vi "Split and merge.vi"(4 "DKE_Meaning":string="'A' leads letters; the Ancient Lord Leads and lords the entire world", 6 "Translation":string="'A' leads letters; the Ancient Lord Leads and lords the entire world", 7 "Index":string="அறத்துப்பால் - பாயிரம் - கடவுள் வாழ்த்து - ", 8 "DKT_Meaning":string="பகவன் முதற்றே உலகு.", 9 "Line 2":string="பகவன் முதற்றே உலகு.", 10 "Line1":string="அகர முதல எழுத்தெல்லாம் ஆதி", 11 "String In":string="\\par\r\n\r\n\\pard\\fi-2880\\li2880\\tx2880\\f2\\lang1097  \\f0  \\par\r\n\\u2990?\\u3009?\\u2965?\\u2984?\\u2965? \\u2984?\\u2975?\\u3021?\\u2986?\\u2980?\\u3009? \\u2984?\\u2975?\\u3021?\\u2986?\\u2985?\\u3021?\\u2993?\\u3009?\\par\r\n\\u2949?\\u2965?\\u2984?\\u2965? \\u2984?\\u2975?\\u3021?\\u2986?\\u2980?\\u3009?\\par\r\n\\b0\\f1\\fs36\\lang1033   \\par\r\nFriendship is not more smile on face\\par\r\nIt is the smiling heart's embrace\\par\r\n\\f2\\fs24\\lang1097   \\f0\\par\r\n\\u2986?\\u3006?\\u2994?\\u3021?- \\u2986?\\u3018?\\u2992?\\u3009?\\u2995?\\u3021?, \\u2951?\\u2991?\\u2994?\\u3021? - \\u2984?\\u2975?\\u3021?\\u2986?\\u3007?\\u2991?\\u2994?\\u3021?, \\u2949?\\u2980?\\u3007?\\u2965?\\u3006?\\u2992?\\u2990?\\u3021? - \\u2984?\\u2975?\\u3021?\\u2986?\\u3009? - ") -> (3 "String Output":string="\\par\r\n\\u2949?\\u2965?\\u2992? \\u2990?\\u3009?\\u2980?\\u2994? \\u2958?\\u2996?\\u3009?\\u2980?\\u3021?\\u2980?\\u3014?\\u2994?\\u3021?\\u2994?\\u3006?\\u2990?\\u3021? \\u2950?\\u2980?\\u3007?\\par\r\n\\u2986?\\u2965?\\u2997?\\u2985?\\u3021? \\u2990?\\u3009?\\u2980?\\u2993?\\u3021?\\u2993?\\u3015? \\u2953?\\u2994?\\u2965?\\u3009?.\\par\r\n\\u2949?\\u2965?\\u2984?\\u2965? \\u2984?\\u2975?\\u3021?\\u2986?\\u2980?\\u3009?\\par\r\n\\b0\\f1\\fs36\\lang1033   \\par\r\n'A' leads letters; the Ancient Lord \\par\r\nLeads and lords the entire world\\par\r\n\\f2\\fs24\\lang1097   \\f0\\par\r\n\\u2949?\\u2993?\\u2980?\\u3021?\\u2980?\\u3009?\\u2986?\\u3021?\\u2986?\\u3006?\\u2994?\\u3021? - \\u2986?\\u3006?\\u2991?\\u3007?\\u2992?\\u2990?\\u3021? - \\u2965?\\u2975?\\u2997?\\u3009?\\u2995?\\u3021? \\u2997?\\u3006?\\u2996?\\u3021?\\u2980?\\u3021?\\u2980?\\u3009? - ")   [LabVIEW 2019]
doc: "This VI is Developed by Anish Prabu T.\n\nCopyright © 2006, email:anishprabu243@yahoo.co.in.\nAll rights reserved."
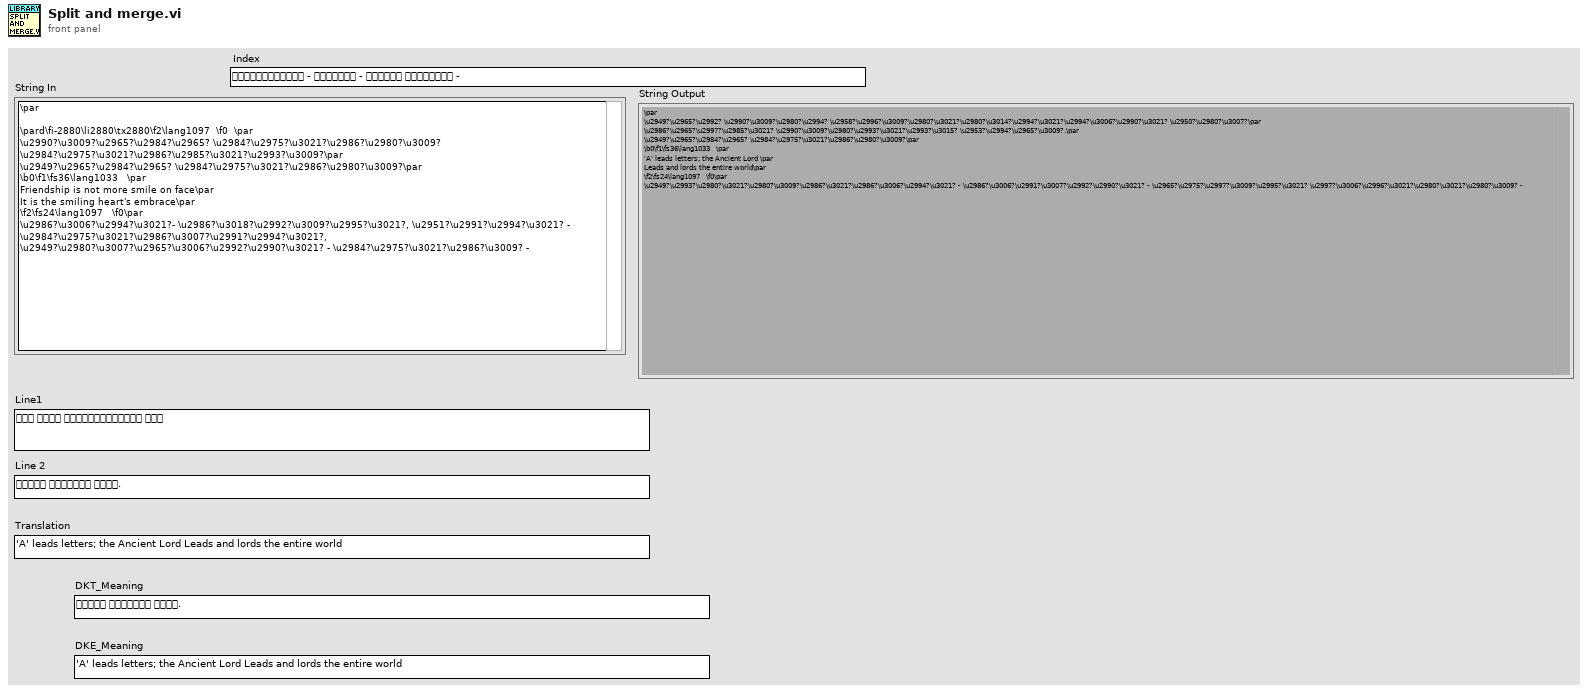
[diagram p1: front panel]
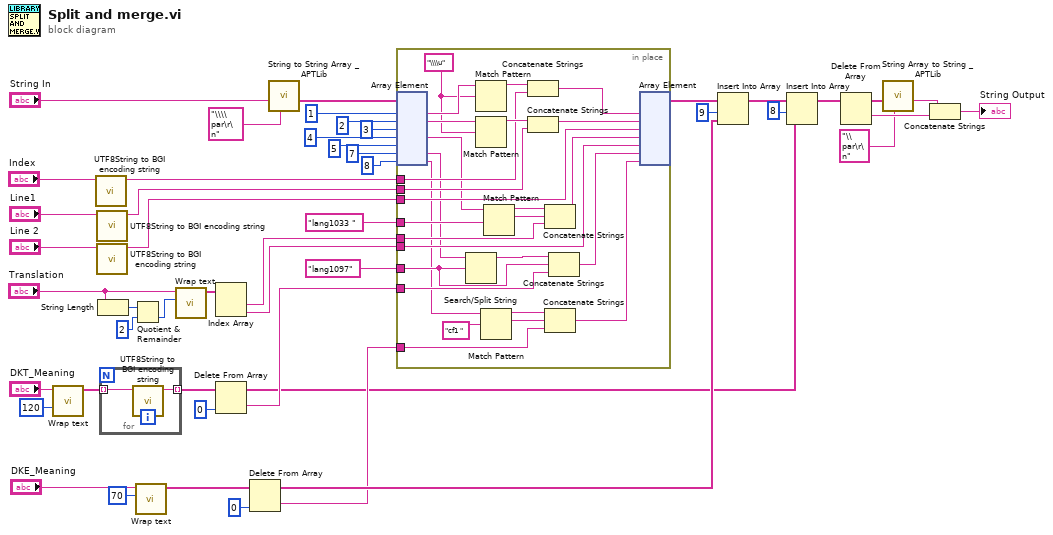
[diagram p0: block diagram]
diagram:
  n1 = call "Wrap text.vi"("Wrap Length"=120, "Text"="DKT_Meaning") -> ("Texts"=w25:string[])  [unwired: 9 in]
  n2 = call "UTF8String to BGI encoding string.vi"("Line1"="Index") -> ("String"=w37:string)  [unwired: 10 in]
  n3 = call "UTF8String to BGI encoding string.vi"("Line1"="Line1") -> ("String"=w35:string)  [unwired: 10 in]
  n4 = call "UTF8String to BGI encoding string.vi"("Line1"="Line 2") -> ("String"=w34:string)  [unwired: 10 in]
  n5 = String Length(string="Translation") -> (length=w12:i32)
  n6 = for {
    tunnel: w25 -> [w50] mode=indexing
    tunnel: [w49] -> w24 mode=indexing
    n7 = call "UTF8String to BGI encoding string.vi"("Line1"=w50) -> ("String"=w49:string)  [unwired: 10 in]
  }
  n8 = Quotient & Remainder(x=w12, y=2) -> (floor(x/y)=w10:i32)  [unwired: 1 out]
  n9 = call "Wrap text.vi"("Wrap Length"=70, "Text"="DKE_Meaning") -> ("Texts"=w14:string[])  [unwired: 9 in]
  n10 = call "Wrap text.vi"("Wrap Length"=w10, "Text"="Translation") -> ("Texts"=w9:string[])  [unwired: 9 in]
  n11 = Index Array(array=w9) -> (element #1=w8:string, element #2=w7:string)  [unwired: 2 in]
  n12 = Delete From Array(array=w24, index=0) -> (deleted portion=w6:string, array with subset deleted=w1:string[])  [unwired: 1 in]
  n13 = Delete From Array(array=w14, index=0) -> (deleted portion=w5:string, array with subset deleted=w18:string[])  [unwired: 1 in]
  n14 = call <userlib>:"String to String Array _APTLib.vi"("Seperator"="\\\\par\r\n", "String Input"="String In") -> ("String Array"=w32:string[])  [unwired: 8 in, 1 out]
  n15 = in-place {
    in-place-border: w37 -> [w69]
    in-place-border: w35 -> [w73]
    in-place-border: w34 -> [w78]
    in-place-border: w8 -> [w63]
    in-place-border: w7 -> [w77]
    in-place-border: w6 -> [w60]
    in-place-border: w5 -> [w56]
    in-place-border: "lang1033 " ("regular expression") -> [w64]
    in-place-border: "lang1097" ("regular expression") -> [w53]
    w68 = "\\\\u" ("regular expression")
    n16 = in-place-array #1(w32, 1, 2 ("index"), 3, 4 ("index"), 5, 7, 8) -> (w72:string, w76:string, w67:string, w55:string, w52:string)  [unwired: 2 out]
    n17 = Search/Split String(string=w55, search string/char (-)=w53) -> (substring before match=w54:string)  [unwired: 1 in, 2 out]
    n18 = Match Pattern(string=w72, regular expression=w68) -> (before substring=w71:string)  [unwired: 1 in, 3 out]
    n19 = Match Pattern(string=w76, regular expression=w68) -> (before substring=w75:string)  [unwired: 1 in, 3 out]
    n20 = Match Pattern(string=w52, regular expression="cf1 ") -> (before substring=w58:string, match substring=w57:string)  [unwired: 1 in, 2 out]
    n21 = Match Pattern(string=w67, regular expression=w64) -> (before substring=w66:string, match substring=w62:string)  [unwired: 1 in, 2 out]
    n22 = Concatenate Strings(w71, w69) -> (w70:string)
    n23 = Concatenate Strings(w75, w73) -> (w74:string)
    n24 = Concatenate Strings(w66, w62, w63) -> (w65:string)
    n25 = Concatenate Strings(w58, w57, w56) -> (w51:string)
    n26 = Concatenate Strings(w54, w53, w60) -> (w61:string)
    n27 = in-place-array #1(w70, w74, w78, w65, w77, w61, w51) -> (w27:string[])  [unwired: 7 out]
  }
  n28 = Insert Into Array(array=w27, index=9, new element=w18) -> (w21:string[])
  n29 = Insert Into Array(array=w21, index=8, new element=w1) -> (w20:string[])
  n30 = Delete From Array(array=w20) -> (deleted portion=w47:string, array with subset deleted=w48:string[])  [unwired: 2 in]
  n31 = call <userlib>:"String Array to String _APTLib.vi"("Seperator"="\\par\r\n", "String Array"=w48) -> ("String Output"=w46:string)  [unwired: 8 in, 1 out]
  n32 = Concatenate Strings(w46, w47) -> (→"String Output":string)
